vi "init.vi"(8 "error in (no error)":errorcluster, 9 "ID query?":bool, 10 "Reset?":bool, 11 "VISA resource name":refnum<visa-resource-name>) -> (0 "error out":errorcluster, 2 "ID string":string, 3 "VISA Refnum out":refnum<visa-resource-name>)   [LabVIEW 2018, in "Aim-TTi CPX400SP.lvlib"]
uses:
  <instrlib>/Aim-TTi CPX400SP/Aim-TTi CPX400SP.lvlib
panel:
  in  "Timeout (ms)":u32=2000
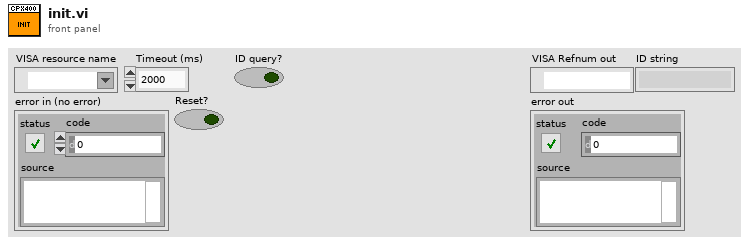
[diagram p1: front panel]
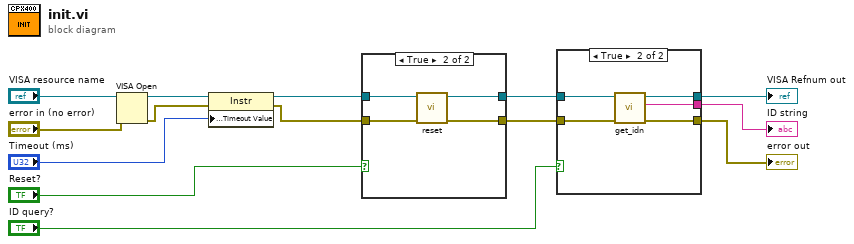
[diagram p0: block diagram]
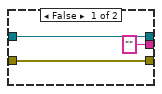
[diagram p2: hidden frame]
diagram:
  n1 = VISA Open(error in (no error)="error in (no error)", VISA resource name="VISA resource name") -> (VISA resource name=w11:refnum<visa-resource-name>, error out=w10:errorcluster)  [unwired: 3 in]
  n2 = property class="Instr"(reference=w11, error in=w10, "General Settings:Timeout Value"="Timeout (ms)") -> (reference out=w7:refnum<visa-resource-name>, error out=w4:errorcluster)
  n3 = case shown="True" "Reset?" {
    tunnel: w7 -> [w16 w20]
    tunnel: [w16 w19] -> w6
    tunnel: [w15 w18] -> w5
    tunnel: w4 -> [w15 w17]
    frame False {
    }
    frame True {
      n4 = call <instrlib>:"reset.vi"("error in (no error)"=w17, "VISA Refnum in"=w20) -> ("error out"=w18:errorcluster, "VISA Refnum out"=w19:refnum<visa-resource-name>)  [unwired: 8 in]
    }
  }
  n5 = case shown="True" "ID query?" {
    tunnel: w6 -> [w23 w28]
    tunnel: w5 -> [w22 w27]
    tunnel: [w23 w26] -> w3
    tunnel: ["" ("idn") w25] -> w1
    tunnel: [w22 w24] -> w2
    frame False {
    }
    frame True {
      n6 = call <instrlib>:"get_idn.vi"("error in (no error)"=w27, "VISA Refnum in"=w28) -> ("error out"=w24:errorcluster, "idn"=w25:string, "VISA Refnum out"=w26:refnum<visa-resource-name>)  [unwired: 7 in]
    }
  }
  "VISA Refnum out" <- w3
  "error out" <- w2
  "ID string" <- w1
